vi "HV Seq Record.vi"() -> ()   [LabVIEW 2017]
doc: "Demonstrates the fundamentals of the Queued Message Handler design pattern in LabVIEW. A queued message handler, in its simplest form, is composed of two loops. The Event Handling Loop responds to user interface events by enqueuing \"messages\" on a message queue. These messages are dequeued in the Message Handling Loop. Note that the Message Handling Loop is also capable of sending messages to itself."
uses:
  Program Files (x86)/National Instruments/LabVIEW 2017/examples/Design Patterns/Queued Message Handler/support/QMH Fundamentals - Message Cluster.ctl
  controls/UI Record Data.ctl
  <vilib>/Utility/error.llb/Error Cluster From Error Code.vi
  <vilib>/ErrorRing/Error Ring.xnode
panel:
  in  "Clear Button":bool
  in  "Next Button":bool
  in  "Previous Button":bool
  in  "Remove Button":bool
  in  "Add Button":bool
  in  "Stop":bool
  out "Current Sequence Step Number":string
  in  "LG Electrodes":bool[][](array[boolean])=[[FALSE, FALSE], [FALSE, FALSE], [FALSE, FALSE]]
  in  "SM Electrodes":bool[][](array[boolean])=[[FALSE, FALSE, FALSE, FALSE, FALSE, FALSE], [FALSE, FALSE, FALSE, FALSE, FALSE, FALSE], [FALSE, FALSE, FALSE, FALSE, FALSE, FALSE], [FALSE, FALSE, FALSE, FALSE, FALSE, FALSE], [FALSE, FALSE, FALSE, FALSE, FALSE, FALSE], [FALSE, FALSE, FALSE, FALSE, FALSE, FALSE]]
  in  "XS Electrodes":bool[][](array[boolean])=[[FALSE, FALSE, FALSE], [FALSE, FALSE, FALSE], [FALSE, FALSE, FALSE], [FALSE, FALSE, FALSE], [FALSE, FALSE, FALSE], [FALSE, FALSE, FALSE]]
  out "Display Message":string
  # "Record Electrode Sequence"
  # "Electrode Controls"
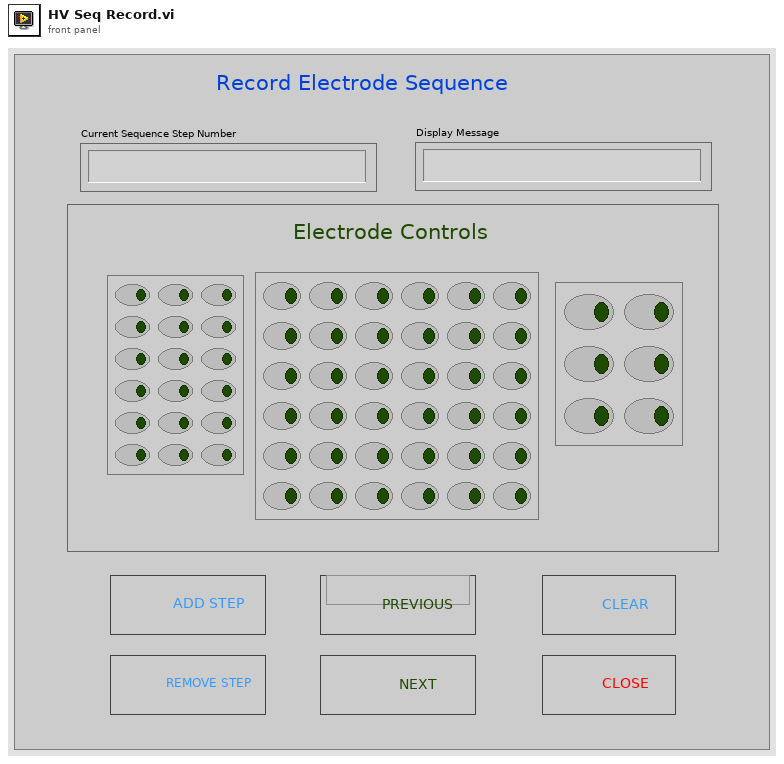
[diagram p1: front panel]
types:
  T1 = typedef "UI Record Data.ctl" = cluster{"Current Sequence Step Number":refnum<vi>, "Display Message":refnum<vi>, "XS Electrodes":refnum<vi>, "SM Electrodes":refnum<vi>, "LG Electrodes":refnum<vi>}
  T2 = typedef "QMH Fundamentals - Message Cluster.ctl" = cluster{"Message":string, "Message Data":variant}
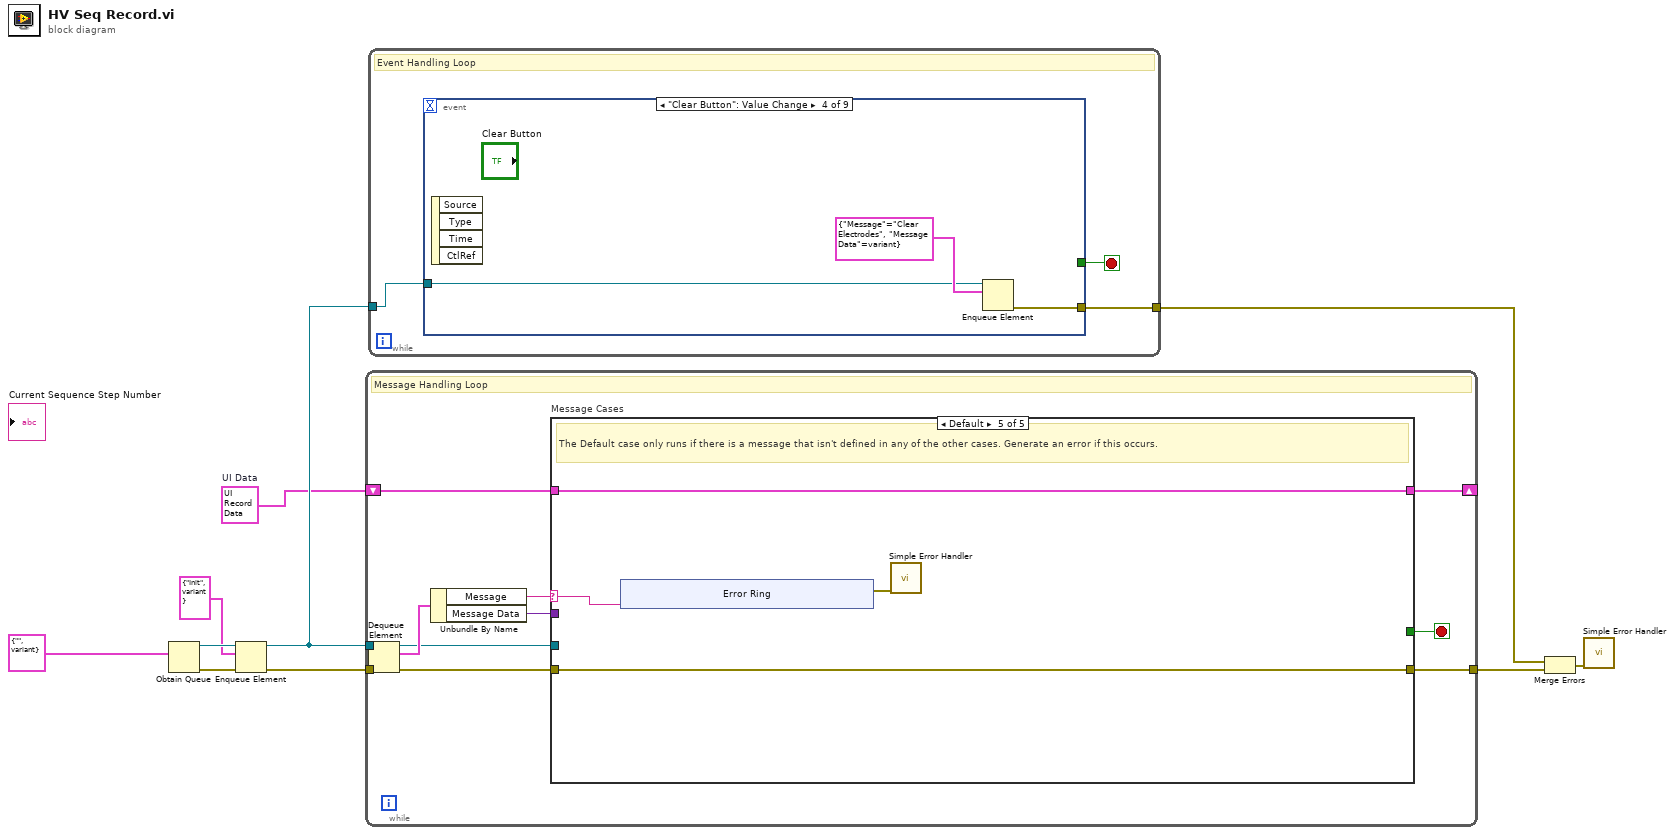
[diagram p0: block diagram]
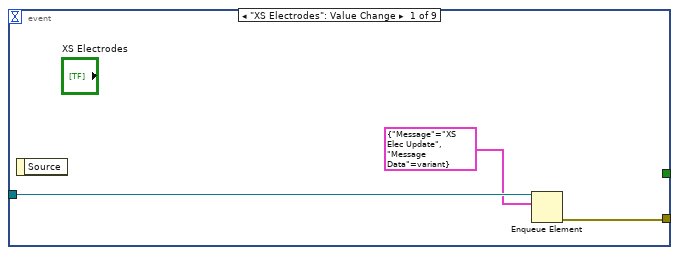
[diagram p2: hidden frame]
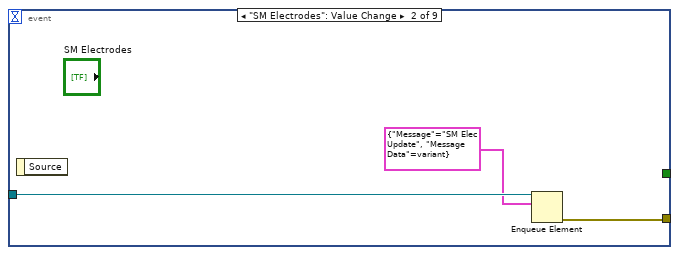
[diagram p3: hidden frame]
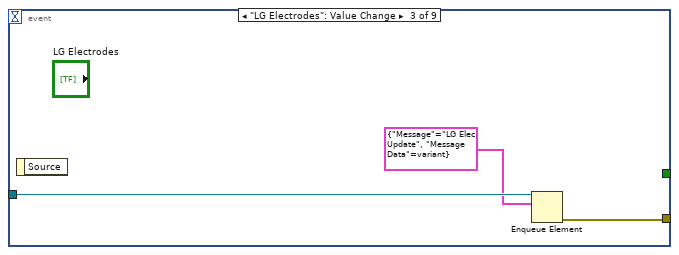
[diagram p4: hidden frame]
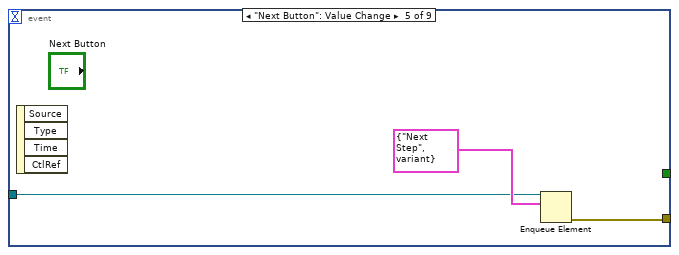
[diagram p5: hidden frame]
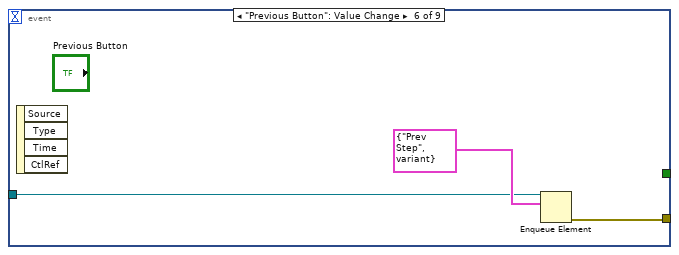
[diagram p6: hidden frame]
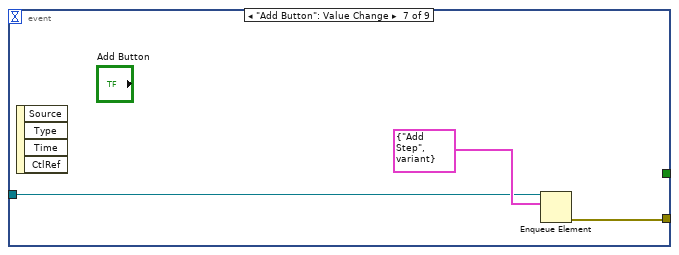
[diagram p7: hidden frame]
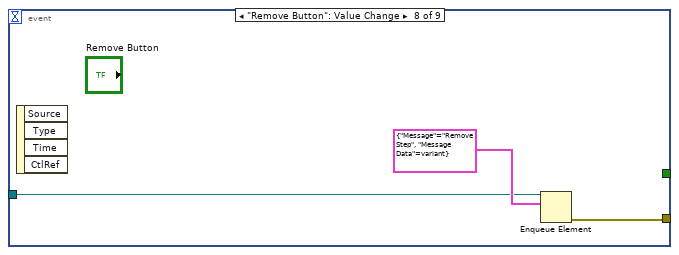
[diagram p8: hidden frame]
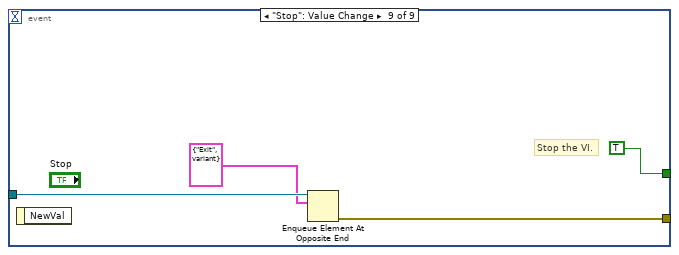
[diagram p9: hidden frame]
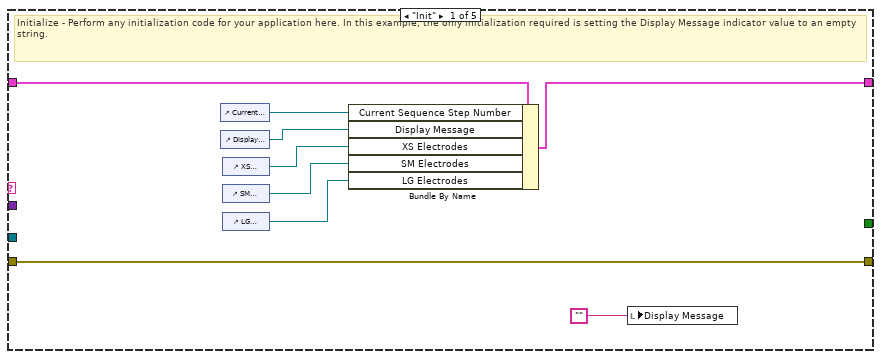
[diagram p10: hidden frame]
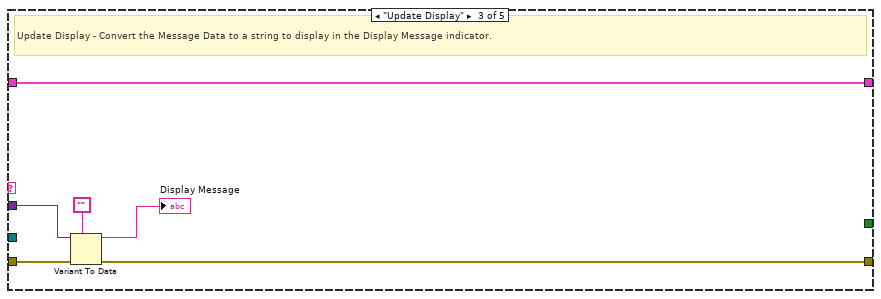
[diagram p12: hidden frame]
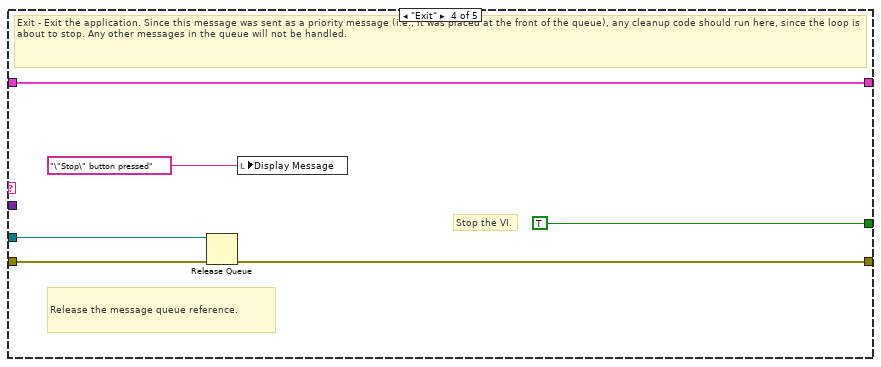
[diagram p13: hidden frame]
diagram:
  w1 = T1 {"Current Sequence Step Number"=refnum, "Display Message"=refnum, "XS Electrodes"=refnum, "SM Electrodes"=refnum, "LG Electrodes"=refnum}  # UI Data
  n1 = Obtain Queue(element data type=T2 {"Message"="", "Message Data"=variant} ("Message Cluster")) -> (queue out=w7:refnum<queue>, error out=w8:errorcluster)  [unwired: 4 in, 1 out]
  n2 = Enqueue Element(queue=w7, element=T2 {"Message"="Init", "Message Data"=variant}, error in (no error)=w8) -> (queue out=w5:refnum<queue>, error out=w6:errorcluster)  [unwired: 1 in, 1 out]
  n3 = while {
    tunnel: w5 -> [w18]
    tunnel: w6 -> [w19]
    tunnel: [w20] -> w10
    shift-right: [w12] -> _
    shift-left: w1 -> [w11]
    stop <- w21 stop-if-true
    # "Message Handling Loop"
    n4 = Dequeue Element(queue=w18, error in (no error)=w19) -> (queue out=w16:refnum<queue>, element=w17:T2, error out=w15:errorcluster)  [unwired: 1 in, 1 out]
    n5 = Unbundle By Name(w17) -> ("Message"=w14:string, "Message Data"=w13:variant)
    n6 = case "Message Cases" shown="Default" w14 {
      selector: w14 -> [_ _ _ _ w48]
      tunnel: w16 -> [_ _ _ w44 _]
      tunnel: w15 -> [w30 w32 w38 w41 w47]
      tunnel: [w30 w32 w35 w42 w47] -> w20
      tunnel: [_ _ _ TRUE _] -> w21
      tunnel: w13 -> [_ _ w37 _ _]
      tunnel: w11 -> [w28 w31 w33 w39 w45]
      tunnel: [w22 w31 w33 w39 w45] -> w12
      frame "Init" {
        # "Initialize - Perform any initialization code for your application here. In this example, the only initialization required is setting the Display Message indicator value to an empty string."
        n7 = control-ref of="Current Sequence Step Number"() -> (w27:refnum<vi>)
        n8 = control-ref of="Display Message"() -> (w26:refnum<vi>)
        n9 = control-ref of="XS Electrodes"() -> (w25:refnum<vi>)
        n10 = control-ref of="SM Electrodes"() -> (w24:refnum<vi>)
        n11 = control-ref of="LG Electrodes"() -> (w23:refnum<vi>)
        n12 = Bundle By Name(cluster=w28, "Current Sequence Step Number"=w27, "Display Message"=w26, "XS Electrodes"=w25, "SM Electrodes"=w24, "LG Electrodes"=w23) -> (w22:T1)
        n13 = local write "Display Message"("") -> ()
      }
      frame "XS Elec Update" {
        # "Update the XS electrode on front panel with new value."
      }
      frame "Update Display" {
        # "Update Display - Convert the Message Data to a string to display in the Display Message indicator."
        n14 = Variant To Data(error in=w38, type="", Variant=w37) -> (data=→"Display Message":string, error out=w35:errorcluster)
      }
      frame "Exit" {
        # "Stop the VI."
        # "Release the message queue reference."
        # "Exit - Exit the application. Since this message was sent as a priority message (i.e., it was placed at the front of the queue), any cleanup code should run here, since the loop is about to stop. Any other messages in the queue will not be handled."
        n15 = Release Queue(queue=w44, error in (no error)=w41) -> (error out=w42:errorcluster)  [unwired: 1 in, 2 out]
        n16 = local write "Display Message"("\"Stop\" button pressed" ("L10n_Stop Pressed")) -> ()
      }
      frame Default {
        # "The Default case only runs if there is a message that isn't defined in any of the other cases. Generate an error if this occurs."
        n17 = xnode "Error Ring"("parameter 0"=w48) -> ("error out"=w46:errorcluster)
        n18 = call <vilib>:"Simple Error Handler.vi"("error in (no error)"=w46) -> ()  [unwired: 4 in, 5 out]
      }
    }
  }
  n19 = while {
    tunnel: w5 -> [w58]
    tunnel: [w56] -> w2
    stop <- w57 stop-if-true
    # "Event Handling Loop"
    n20 = event shown="[3] \"Clear Button\": Value Change" {
      selector: _ -> [_ _ _ _ _ _ _ _ _]
      dyn-events: _ -> [_ _ _ _ _ _ _ _ _]
      timeout: _ -> [_ _ _ _ _ _ _ _ _]
      tunnel: [_ _ _ _ _ _ _ _ TRUE] -> w57
      tunnel: w58 -> [w60 w63 w66 w68 w71 w74 w77 w80 w86]
      tunnel: [w61 w64 w67 w69 w72 w75 w78 w81 w85] -> w56
      event "XS Electrodes": Value Change {
        n21 = event-data() -> ()  [unwired: 1 in, 1 out]
        n22 = Enqueue Element(queue=w60, element=T2 {"Message"="XS Elec Update", "Message Data"=variant}) -> (error out=w61:errorcluster)  [unwired: 2 in, 2 out]
      }
      event "SM Electrodes": Value Change {
        n23 = event-data() -> ()  [unwired: 1 in, 1 out]
        n24 = Enqueue Element(queue=w63, element=T2 {"Message"="SM Elec Update", "Message Data"=variant}) -> (error out=w64:errorcluster)  [unwired: 2 in, 2 out]
      }
      event "LG Electrodes": Value Change {
        n25 = event-data() -> ()  [unwired: 1 in, 1 out]
        n26 = Enqueue Element(queue=w66, element=T2 {"Message"="LG Elec Update", "Message Data"=variant}) -> (error out=w67:errorcluster)  [unwired: 2 in, 2 out]
      }
      event "Clear Button": Value Change {
        n27 = event-data() -> ()  [unwired: 1 in, 4 out]
        n28 = Enqueue Element(queue=w68, element=T2 {"Message"="Clear Electrodes", "Message Data"=variant}) -> (error out=w69:errorcluster)  [unwired: 2 in, 2 out]
      }
      event "Next Button": Value Change {
        n29 = event-data() -> ()  [unwired: 1 in, 4 out]
        n30 = Enqueue Element(queue=w71, element=T2 {"Message"="Next Step", "Message Data"=variant}) -> (error out=w72:errorcluster)  [unwired: 2 in, 2 out]
      }
      event "Previous Button": Value Change {
        n31 = event-data() -> ()  [unwired: 1 in, 4 out]
        n32 = Enqueue Element(queue=w74, element=T2 {"Message"="Prev Step", "Message Data"=variant}) -> (error out=w75:errorcluster)  [unwired: 2 in, 2 out]
      }
      event "Add Button": Value Change {
        n33 = event-data() -> ()  [unwired: 1 in, 4 out]
        n34 = Enqueue Element(queue=w77, element=T2 {"Message"="Add Step", "Message Data"=variant}) -> (error out=w78:errorcluster)  [unwired: 2 in, 2 out]
      }
      event "Remove Button": Value Change {
        n35 = event-data() -> ()  [unwired: 1 in, 4 out]
        n36 = Enqueue Element(queue=w80, element=T2 {"Message"="Remove Step", "Message Data"=variant}) -> (error out=w81:errorcluster)  [unwired: 2 in, 2 out]
      }
      event "Stop": Value Change {
        # "Stop the VI."
        # "Enqueue an \"Exit\" message. Note that the Enqueue Element At Opposite End function is used to place this priority \"Exit\" message at the front of the queue ahead of all other messages."
        n37 = event-data() -> ()  [unwired: 1 in, 1 out]
        n38 = Enqueue Element At Opposite End(queue=w86, element=T2 {"Message"="Exit", "Message Data"=variant}) -> (error out=w85:errorcluster)  [unwired: 2 in, 2 out]
      }
    }
  }
  n39 = Merge Errors(w2, w10) -> (w3:errorcluster)
  n40 = call <vilib>:"Simple Error Handler.vi"("error in (no error)"=w3) -> ()  [unwired: 4 in, 5 out]
